vi "central difference (i32).vi"(3 "Y":i32[](array[numeric])) -> (5 "0.5*(Y(i+1)-Y(i-1))":i32[](array[numeric]))   [LabVIEW 2009, in "common.lvlib"]
uses:
  common.lvlib
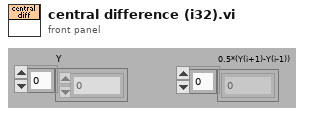
[diagram p1: front panel]
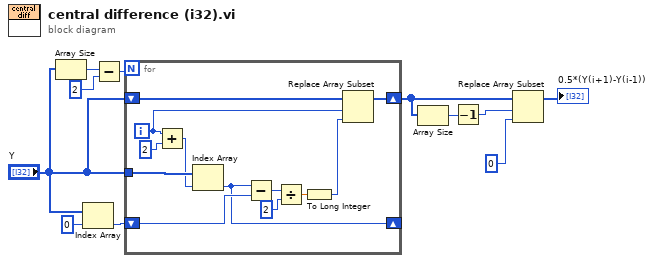
[diagram p0: block diagram]
diagram:
  n1 = Array Size(array="Y") -> (size(s)=w3:i32)
  n2 = Index Array(array="Y", index=0) -> (element=w10:i32)
  n3 = Subtract(x=w3, y=2 ("size(s)")) -> (x-y=w2:i32)
  n4 = for {
    N: w2 -> [_]
    tunnel: "Y" -> [w23]
    shift-right: [w20] -> _
    shift-left: w10 -> [w21]
    shift-right: [w18] -> w7
    shift-left: "Y" -> [w19]
    i -> [w17]
    n5 = Add(x=w17, y=2 ("size(s)")) -> (x+y=w22:i32)
    n6 = Index Array(array=w23, index=w22) -> (element=w20:i32)
    n7 = Subtract(x=w20, y=w21) -> (x-y=w15:i32)
    n8 = Divide(x=w15, y=2 ("size(s)")) -> (x/y=w13:dbl)
    n9 = To Long Integer(number=w13) -> (32bit integer=w12:i32)
    n10 = Replace Array Subset(array=w19, new element=w12, index=w17) -> (w18:i32[])
  }
  n11 = Array Size(array=w7) -> (size(s)=w6:i32)
  n12 = Decrement(x=w6) -> (x-1=w5:i32)
  n13 = Replace Array Subset(array=w7, new element=0 ("new element/subarray"), index=w5) -> (→"0.5*(Y(i+1)-Y(i-1))":i32[])
